vi "update config.vi"(8 "error in (no error)":errorcluster, 10 "user configurations":T1={"vst_device"=["VST_1", "VST_2"], "RF gain "=10.0, "buffer size"=524288, "center frequency (Hz) "=1000000000.0, "P2P sample rate"=200000000.0, "mode"=enum."5785 - 2*180MHz", "devicess"=["IF_transiver_0", "IF_transiver_1", "IF_transiver_2"], "gen for df"=FALSE, "Rx settings"={"min PW         "=0.0, "max gap        "=0.0, "detection bar"=0.0, "peak detect                        "=FALSE}}, 11 "5785_2_X_400MHz_Rx_as_scop in":refnum<class "5785_2_X_400MHz_Rx_as_scop.lvclass">) -> (0 "error out":errorcluster, 1 "min frequency":dbl, 2 "max frequency":dbl, 3 "5785_2_X_400MHz_Rx_as_scop out":refnum<class "5785_2_X_400MHz_Rx_as_scop.lvclass">)   [LabVIEW 2021, in "5785_2_X_400MHz_Rx_as_scop.lvclass"]
uses:
  5785_2_X_400MHz_Rx_as_scop.lvclass
  pulse_tx_vis/CTL/user config.ctl
  <vilib>/userdefined/High Color/nirio_resource_hc.ctl
  5785_2_X_400MHz_Rx_as_scop.lvclass/5785_2_X_400MHz_Rx_as_scop.ctl
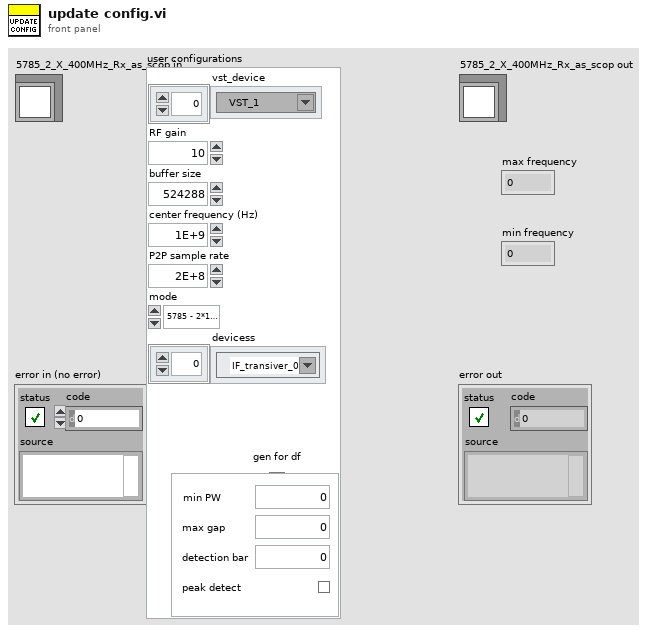
[diagram p1: front panel]
types:
  T1 = typedef "user config.ctl" = cluster{"vst_device":refnum<k15>[], "RF gain ":dbl, "buffer size":u32, "center frequency (Hz) ":dbl, "P2P sample rate":dbl, "mode":enum16{"USRP - 180MHz", "5785 - 2*180MHz", "5785 - 3.2GHz", "P2P - VST"}, "devicess":T2[], "gen for df":bool, "Rx settings":cluster{"min PW         ":dbl, "max gap        ":dbl, "detection bar":dbl, "peak detect                        ":bool}}
  T2 = typedef "nirio_resource_hc.ctl" = tag
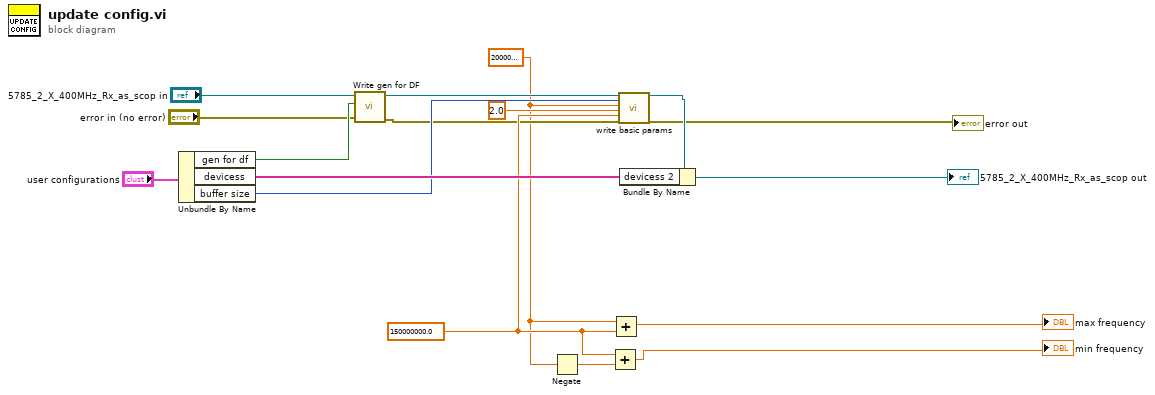
[diagram p0: block diagram]
diagram:
  w13 = 150000000.0
  w1 = 200000000.0 ("Fs  FPGA")
  n1 = Unbundle By Name("user configurations") -> ("gen for df"=w10:bool, "devicess"=w17:T2[], "buffer size"=w15:u32)
  n2 = call-dynamic "Write gen for DF.vi"("error in (no error)"="error in (no error)", "gen for DF"=w10, "device_type in"="5785_2_X_400MHz_Rx_as_scop in") -> ("error out"=w9:errorcluster, "device_type out"=w11:refnum<class "5785_2_X_400MHz_Rx_as_scop.lvclass">)  [unwired: 7 in]
  n3 = Negate(x=w1) -> (-x=w16:dbl)
  n4 = Add(x=w13, y=w16) -> (x+y=→"min frequency":dbl)
  n5 = Add(x=w1, y=w13) -> (x+y=→"max frequency":dbl)
  n6 = call-dynamic "write basic params.vi"("device_type in"=w11, "buffer size"=w15, "Fs  FPGA"=w1, "SPC"=2.0 ("Fs  FPGA"), "center frequency (Hz)"=w13, "error in (no error)"=w9) -> ("device_type out"=w12:refnum<class "5785_2_X_400MHz_Rx_as_scop.lvclass">, "error out"=→"error out":errorcluster)  [unwired: 12 in]
  n7 = Bundle By Name(cluster=w12, "devicess 2"=w17) -> (→"5785_2_X_400MHz_Rx_as_scop out":refnum<class "5785_2_X_400MHz_Rx_as_scop.lvclass">)
